vi "parse file scan single scan.vi"(7 "command":bool, 8 "error in (no error)":errorcluster, 9 "values and # shots":string, 10 "variables":string, 11 "Devices":string) -> (0 "error out":errorcluster, 1 "States Out":string, 2 "Variables []":string[](array[string]), 3 "Devices []":string[](array[string]), 4 "Bin #s":i32[](array[numeric]), 5 "values and # shots []":string[](array[string]), 6 "first scan cmd":string)   [LabVIEW 2020]
uses:
  <vilib>/regexp/Match Regular Expression.xnode
panel:
  in  "States in":string
  # "StartScan\ncmd>>dev1>>var1>>val1\nfire\nfire\nfire"
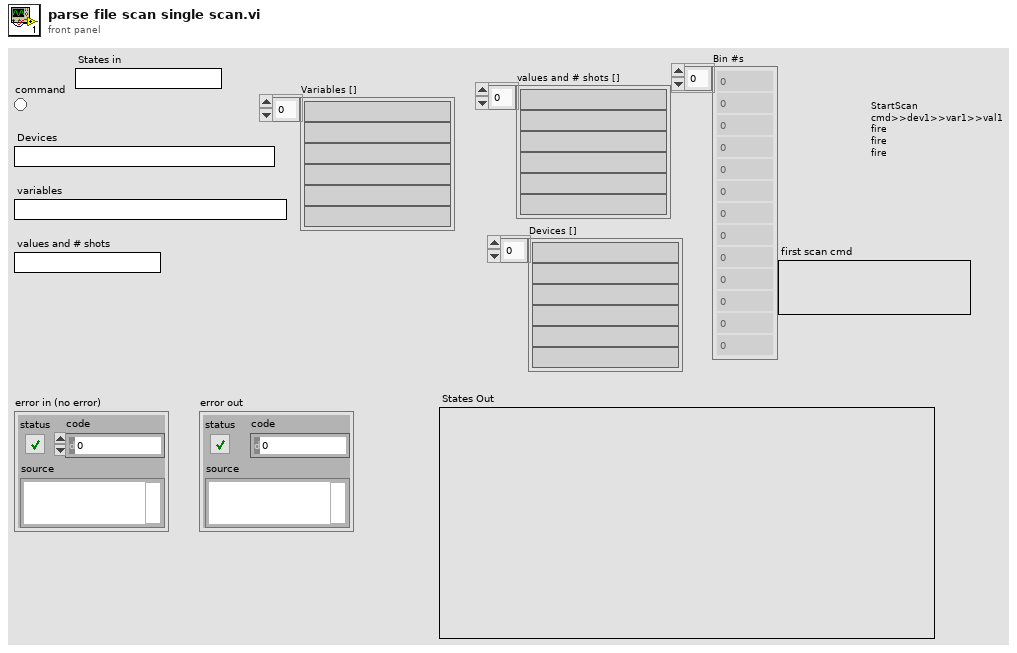
[diagram p1: front panel]
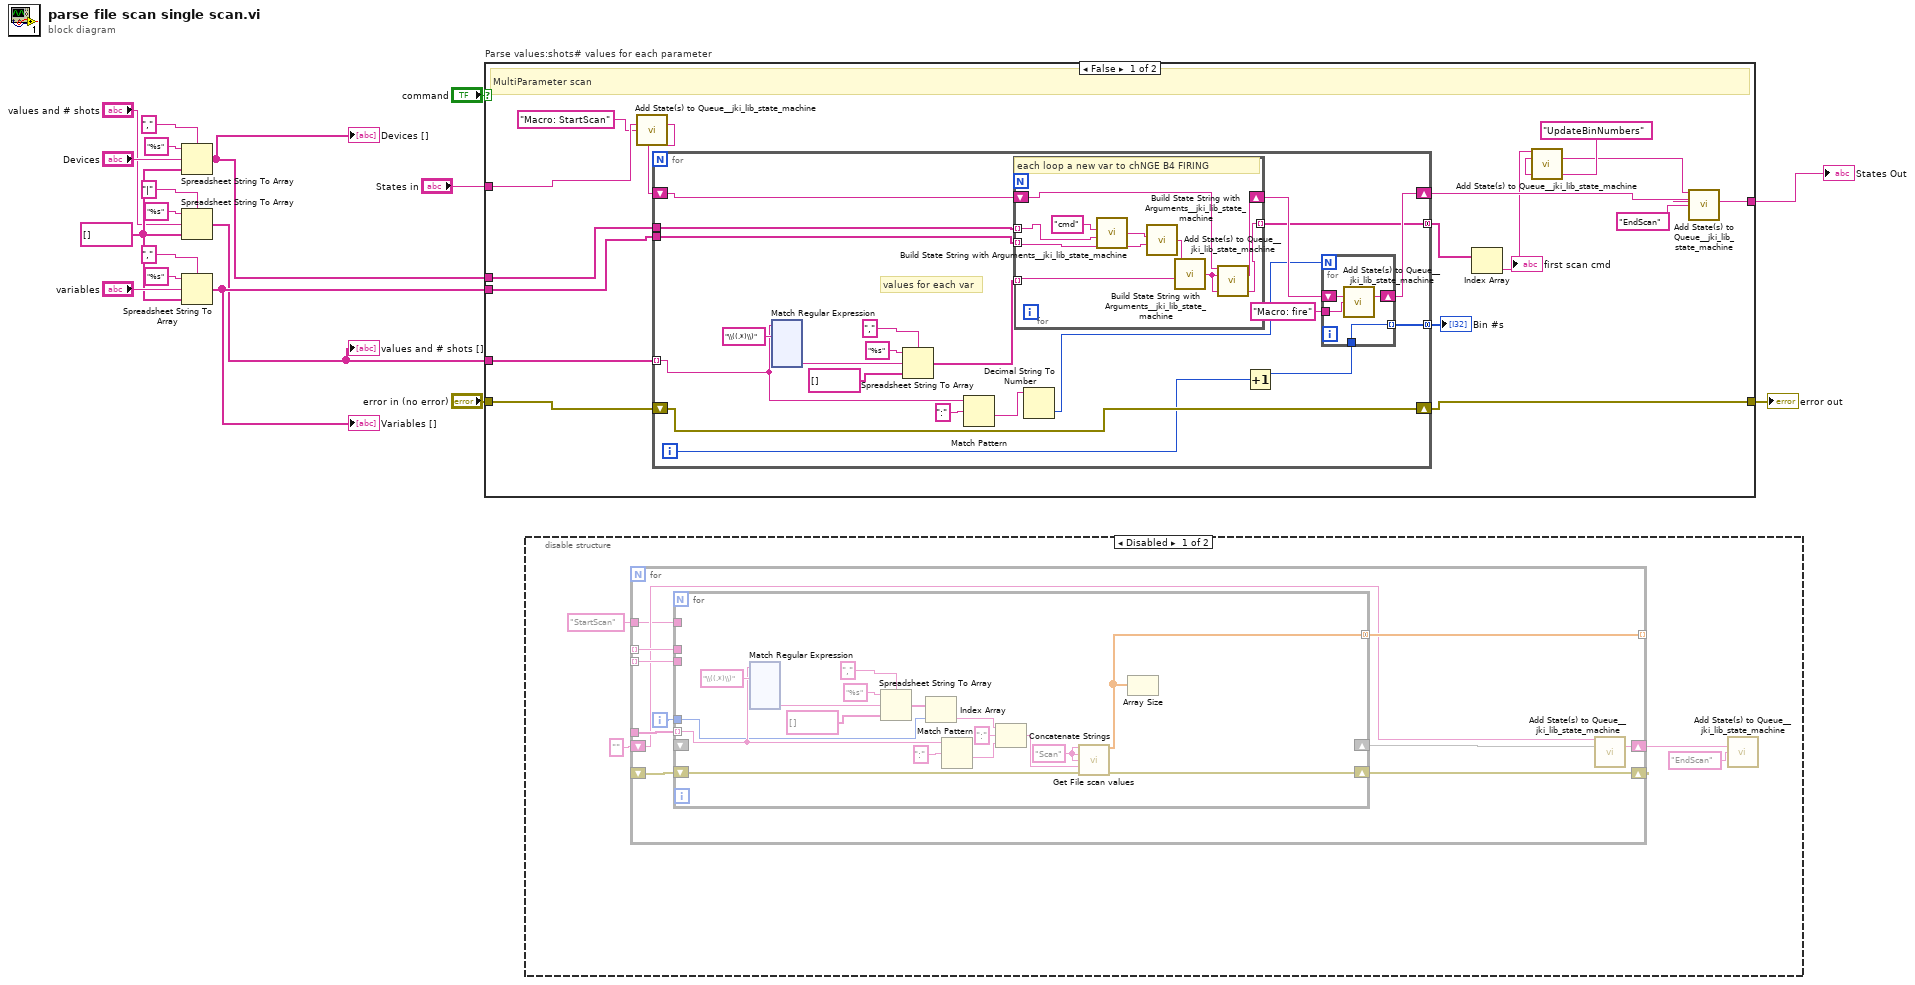
[diagram p0: block diagram]
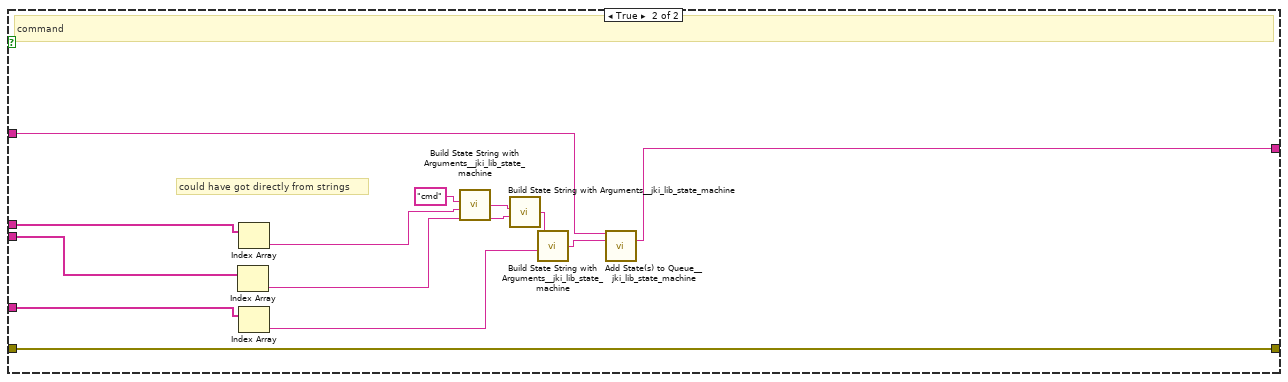
[diagram p3: hidden frame]
diagram:
  w4 = string[] []
  n1 = Spreadsheet String To Array(delimiter (Tab)=",", format string="%s", spreadsheet string="Devices", array type (2D Dbl)=w4) -> (array=w14:string[])
  "Devices []" <- w14
  n2 = Spreadsheet String To Array(delimiter (Tab)="|", format string="%s", spreadsheet string="values and # shots", array type (2D Dbl)=w4) -> (array=w5:string[])
  "values and # shots []" <- w5
  n3 = Spreadsheet String To Array(delimiter (Tab)=",", format string="%s", spreadsheet string="variables", array type (2D Dbl)=w4) -> (array=w16:string[])
  "Variables []" <- w16
  n4 = case "Parse values:shots# values for each parameter" shown="False" "command" {
    tunnel: w5 -> [w34 w188]
    tunnel: "error in (no error)" -> [w33 w197]
    tunnel: [w32 w197] -> w15
    tunnel: w14 -> [w31 w192]
    tunnel: w16 -> [w30 w191]
    tunnel: [w27 w185] -> w18
    tunnel: "States in" -> [w21 w186]
    frame False {
      # "MultiParameter scan"
      n5 = call <vilib>:"Add State(s) to Queue__jki_lib_state_machine.vi"("State(s) in (\"\")"=w21, "State(s) at Back (\"\")"="Macro: StartScan" ("State(s) at Back (\"\")")) -> ("States Out"=w19:string)  [unwired: 13 in]
      n6 = for {
        tunnel: w34 -> [w49] mode=indexing
        shift-right: [w40] -> w32
        shift-left: w33 -> [w40]
        tunnel: w31 -> [w48]
        tunnel: w30 -> [w47]
        shift-right: [w43] -> w29
        shift-left: w19 -> [w41]
        tunnel: [w38] -> w26 mode=concatenating
        tunnel: [w35] -> w25 mode=concatenating
        i -> [w36]
        # "values for each var"
        n7 = xnode "Match Regular Expression"("input string"=w49, "regular expression"="\\((.*)\\)") -> ("submatch 1"=w53:string)  [unwired: 4 in, 5 out]
        n8 = Spreadsheet String To Array(delimiter (Tab)=",", format string="%s", spreadsheet string=w53, array type (2D Dbl)=string[] []) -> (array=w46:string[])
        n9 = Match Pattern(string=w49, regular expression=":") -> (after substring=w45:string)  [unwired: 1 in, 3 out]
        n10 = for {
          tunnel: w48 -> [w65] mode=indexing
          tunnel: w47 -> [w64] mode=indexing
          tunnel: w46 -> [w63] mode=indexing
          shift-right: [w61] -> w42
          shift-left: w41 -> [w62]
          tunnel: [w60] -> w35 mode=indexing
          # "each loop a new var to chNGE B4 FIRING"
          n11 = call <vilib>:"Build State String with Arguments__jki_lib_state_machine.vi"("Arguments (\"\")"=w65, "State"="cmd") -> ("State with Arguments"=w67:string)  [unwired: 4 in]
          n12 = call <vilib>:"Build State String with Arguments__jki_lib_state_machine.vi"("Arguments (\"\")"=w64, "State"=w67) -> ("State with Arguments"=w68:string)  [unwired: 4 in]
          n13 = call <vilib>:"Build State String with Arguments__jki_lib_state_machine.vi"("Arguments (\"\")"=w63, "State"=w68) -> ("State with Arguments"=w60:string)  [unwired: 4 in]
          n14 = call <vilib>:"Add State(s) to Queue__jki_lib_state_machine.vi"("State(s) in Front (\"\")"=w62, "State(s) in (\"\")"=w60) -> ("States Out"=w61:string)  [unwired: 13 in]
        }
        n15 = Decimal String To Number(string=w45) -> (number=w39:i32)  [unwired: 2 in, 1 out]
        n16 = Increment(x=w36) -> (x+1=w37:i32)
        n17 = for {
          N: w39 -> [_]
          shift-right: [w57] -> w43
          shift-left: w42 -> [w58]
          tunnel: "Macro: fire" ("Scan/Command") -> [w59]
          tunnel: w37 -> [w56]
          tunnel: [w56] -> w38 mode=indexing
          n18 = call <vilib>:"Add State(s) to Queue__jki_lib_state_machine.vi"("State(s) in (\"\")"=w58, "State(s) at Back (\"\")"=w59) -> ("States Out"=w57:string)  [unwired: 13 in]
        }
      }
      "Bin #s" <- w26
      n19 = Index Array(array=w25) -> (element=w24:string)  [unwired: 1 in]
      "first scan cmd" <- w24
      n20 = call <vilib>:"Add State(s) to Queue__jki_lib_state_machine.vi"("State(s) in Front (\"\")"=w24, "State(s) in (\"\")"="UpdateBinNumbers" ("State(s) in Front (\"\")")) -> ("States Out"=w22:string)  [unwired: 13 in]
      n21 = call <vilib>:"Add State(s) to Queue__jki_lib_state_machine.vi"("State(s) in Front (\"\")"=w22, "State(s) in (\"\")"=w29, "State(s) at Back (\"\")"="EndScan" ("State(s) at Back (\"\")")) -> ("States Out"=w27:string)  [unwired: 12 in]
    }
    frame True {
      # "could have got directly from strings"
      # "command"
      n22 = Index Array(array=w191) -> (element=w189:string)  [unwired: 1 in]
      n23 = Index Array(array=w192) -> (element=w190:string)  [unwired: 1 in]
      n24 = Index Array(array=w188) -> (element=w187:string)  [unwired: 1 in]
      n25 = call <vilib>:"Build State String with Arguments__jki_lib_state_machine.vi"("Arguments (\"\")"=w190, "State"="cmd") -> ("State with Arguments"=w194:string)  [unwired: 4 in]
      n26 = call <vilib>:"Build State String with Arguments__jki_lib_state_machine.vi"("Arguments (\"\")"=w189, "State"=w194) -> ("State with Arguments"=w195:string)  [unwired: 4 in]
      n27 = call <vilib>:"Build State String with Arguments__jki_lib_state_machine.vi"("Arguments (\"\")"=w187, "State"=w195) -> ("State with Arguments"=w196:string)  [unwired: 4 in]
      n28 = call <vilib>:"Add State(s) to Queue__jki_lib_state_machine.vi"("State(s) in Front (\"\")"=w186, "State(s) in (\"\")"=w196) -> ("States Out"=w185:string)  [unwired: 13 in]
    }
  }
  "States Out" <- w18
  "error out" <- w15
  n29 = disable-structure shown="Disabled" {
    frame Disabled {
      n30 = for {
        tunnel: [w218] -> w198
        tunnel: [w217] -> w199 mode=indexing
        shift-right: [w215] -> w201
        shift-left: [w216] -> w200
        tunnel: [w213] -> w202 mode=indexing
        tunnel: [w212] -> w203 mode=indexing
        shift-right: [w211] -> w206
        shift-left: "" ("States Out") -> [w210]
        tunnel: "StartScan" ("Scan/Command") -> [w208]
        i -> [w214]
        n31 = for {
          tunnel: w218 -> [w229] mode=indexing
          tunnel: [w222] -> w217 mode=concatenating
          shift-right: [w226] -> w215
          shift-left: w216 -> [w225]
          tunnel: w214 -> [w224]
          tunnel: w213 -> [w220]
          tunnel: w212 -> [w219]
          shift-right: [_] -> w209
          shift-left: _ -> [_]
          tunnel: w208 -> [_]
          w227 = "Scan" ("Scan/Command")
          n32 = xnode "Match Regular Expression"("input string"=w229, "regular expression"="\\((.*)\\)") -> ("submatch 1"=w236:string)  [unwired: 4 in, 5 out]
          n33 = Spreadsheet String To Array(delimiter (Tab)=",", format string="%s", spreadsheet string=w236, array type (2D Dbl)=string[] []) -> (array=w235:string[])
          n34 = Index Array(array=w235, index=w224) -> (element=w234:string)
          n35 = Match Pattern(string=w229, regular expression=":") -> (after substring=w231:string)  [unwired: 1 in, 3 out]
          n36 = Concatenate Strings(w234, ":" ("string"), w231) -> (w228:string)
          n37 = call "Get File scan values.vi"("Device"=w227, "Variable"=w227, "Scan/Command"=w227, "Values: Shots#"=w228, "error in (no error)"=w225) -> ("File scan values"=w222:dbl[], "values"=w221:string[], "error out"=w226:errorcluster)  [unwired: 8 in]
          n38 = Array Size(array=w222) -> (size(s)=w223:i32)
        }
        n39 = call <vilib>:"Add State(s) to Queue__jki_lib_state_machine.vi"("State(s) in Front (\"\")"=w210, "State(s) in (\"\")"=w209) -> ("States Out"=w211:string)  [unwired: 13 in]
      }
      n40 = call <vilib>:"Add State(s) to Queue__jki_lib_state_machine.vi"("State(s) in (\"\")"=w206, "State(s) at Back (\"\")"="EndScan" ("Scan/Command")) -> ()  [unwired: 13 in, 1 out]
    }
    frame Enabled {
    }
  }
